vi "Begin.vi"(8 "error in":errorcluster) -> (0 "error out":errorcluster)   [LabVIEW 2023]
doc: "Called before other user functions, this VI is expected to open initial I/O refnums, load in file data, and do all program initialization. Notice that the <B>error out</B> terminal is simply used for data flow. Wiring it to other structures or subVIs ensures that this VI runs first."
uses:
  <vilib>/Rock Robotics/WPI/DriverStation/WPI_DriverStationRobotMode2.ctl
  <vilib>/Rock Robotics/WPI/Joystick/WPI_JoystickDeviceEnum.ctl
  <vilib>/Rock Robotics/WPI/RobotDrive/WPI_RobotDriveDevRef.ctl
  <vilib>/Rock Robotics/WPI/MotorControl/WPI_MotorControlDeviceRef.ctl
  <vilib>/Rock Robotics/WPI/MotorControl/WPI_MotorControlType.ctl
  <vilib>/Rock Robotics/SystemInterfaces/DIO/FPGA_DIOPWMChannel.ctl
  <vilib>/Rock Robotics/WPI/PWM/WPI_PWMDeadband.ctl
  <vilib>/Rock Robotics/SystemInterfaces/DIO/FPGA_DIOChannel.ctl
  <vilib>/Rock Robotics/WPI/SafetyOutput/WPI_SafetyOutputConfigMenu.ctl
  Robot Global Data.vi
  <vilib>/Rock Robotics/Network Tables/NT Write String Array.vi
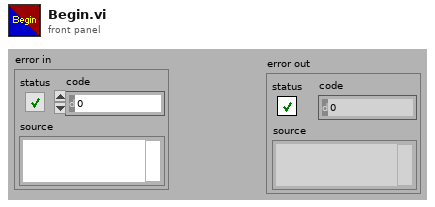
[diagram p1: front panel]
types:
  T1 = typedef "WPI_RobotDriveDevRef.ctl" = cluster{"DevStatus":errorcluster, "Motors[]":T2[], "Square Inputs":bool, "Max Output":dbl}
  T2 = typedef "WPI_MotorControlDeviceRef.ctl" = cluster{"DeviceStatus":errorcluster, "Type":T3, "PWM":cluster{"PWM Channel":T4, "DeadBand":T5}, "CAN":cluster{"Device Number":u8, "SetOutput VI Ref":variant, "GetOutput VI Ref":variant, "Enable VI Ref":variant, "Disable VI Ref":variant, "Data":variant}, "Invert":bool, "DIO PWM":cluster{"PWM \"Enable\" Channel":T4, "DIOChannel":T6, "PWM Rate":dbl}}
  T3 = typedef "WPI_MotorControlType.ctl" = enum16{"PWM", "CAN", "DIO PWM"}
  T4 = typedef "FPGA_DIOPWMChannel.ctl" = enum8{"PWM 0", "PWM 1", "PWM 2", "PWM 3", "PWM 4", "PWM 5", "PWM 6", "PWM 7", "PWM 8", "PWM 9", "PWM MXP 0", "PWM MXP 1", "PWM MXP 2", "PWM MXP 3", "PWM MXP 4", "PWM MXP 5", "PWM MXP 6", "PWM MXP 7", "PWM MXP 8", "PWM MXP 9", "Invalid"}
  T5 = typedef "WPI_PWMDeadband.ctl" = cluster{"Name":string, "maxPositivePwm":i32, "minPositivePwm":i32, "centerPwm":i32, "maxNegativePwm":i32, "minNegativePwm":i32, "angularRange":u16}
  T6 = typedef "FPGA_DIOChannel.ctl" = enum8{"DIO 0", "DIO 1", "DIO 2", "DIO 3", "DIO 4", "DIO 5", "DIO 6", "DIO 7", "DIO 8", "DIO 9", "DIO MXP 0", "DIO MXP 1", "DIO MXP 2", "DIO MXP 3", "DIO MXP 4", "DIO MXP 5", "DIO MXP 6", "DIO MXP 7", "DIO MXP 8", "DIO MXP 9", "DIO MXP 10", "DIO MXP 11", "DIO MXP 12", "DIO MXP 13", "DIO MXP 14", "DIO MXP 15", "SPI Port CS1", "SPI Port CS2", "SPI Port CS3", "SPI Port MISO", "SPI Port MOSI", "Invalid"}
  T7 = typedef "WPI_SafetyOutputConfigMenu.ctl" = enum16{"Enable", "Disable"}
  T8 = typedef "WPI_JoystickDeviceEnum.ctl" = enum16{"USB 0", "USB 1", "USB 2", "USB 3", "USB 4", "USB 5"}
  T9 = typedef "WPI_DriverStationRobotMode2.ctl" = enum16{"Autonomous Disabled", "Autonomous Enabled", "Teleop Disabled", "Teleop Enabled", "Disconnected", "Finish", "Test Disabled", "Test Enabled", "Emergency Stopped"}
  T10 = typedef "WPI_JoystickDevRef.ctl" = cluster{"Device":T8}
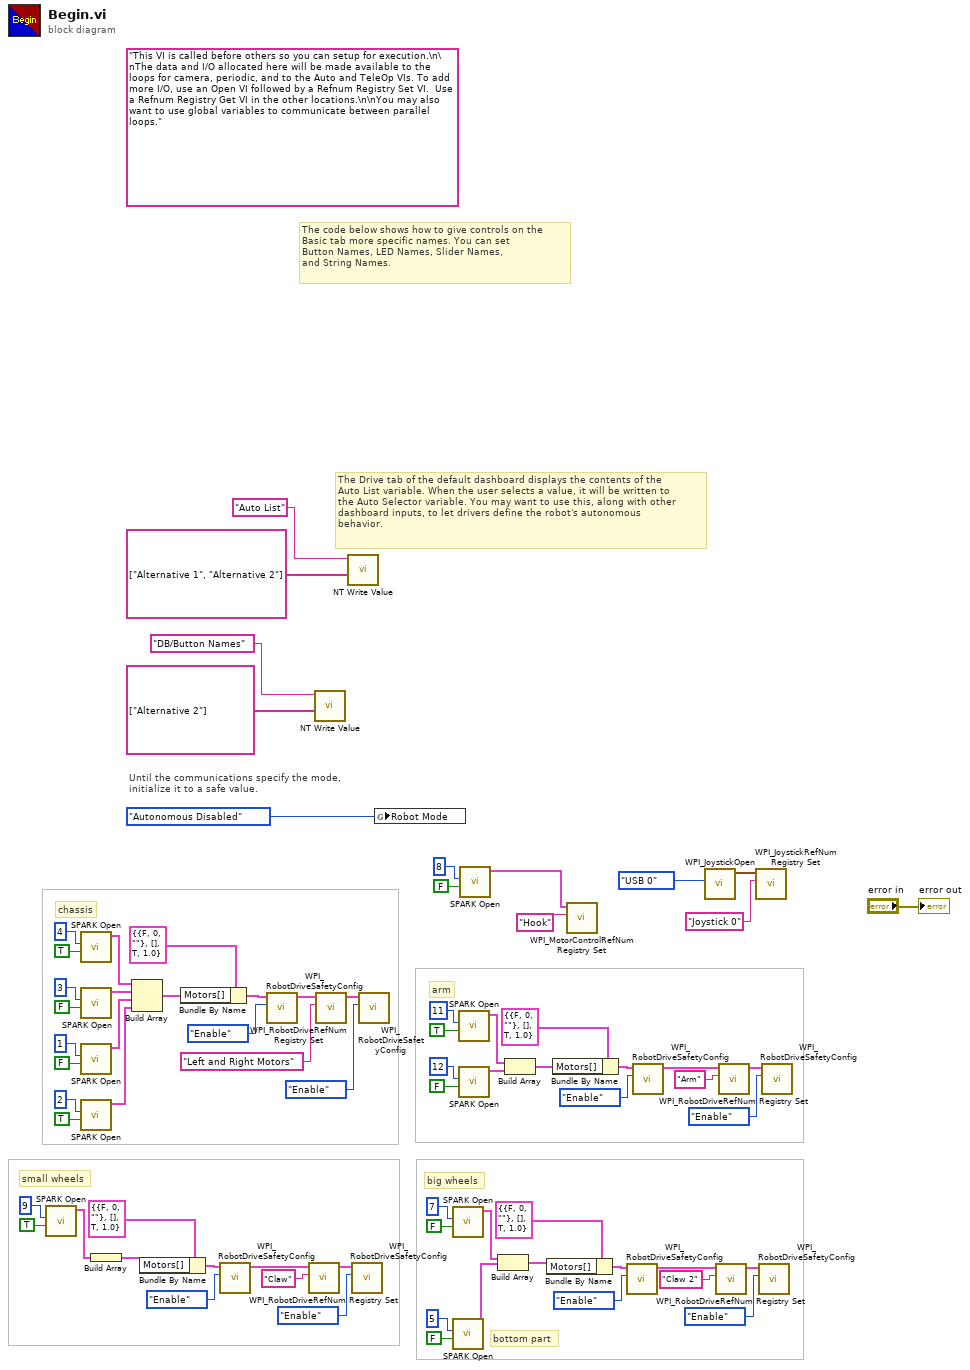
[diagram p0: block diagram]
diagram:
  (unwired) "This VI is called before others so you can setup for execution.\n\nThe data and I/O allocated here will be made available to the loops for camera, periodic, and to the Auto and TeleOp VIs. To add more I/O, use an Open VI followed by a Refnum Registry Set VI.  Use a Refnum Registry Get VI in the other locations.\n\nYou may also want to use global variables to communicate between parallel loops."
  # "bottom part"
  # "arm"
  # "small wheels"
  # "big wheels"
  # "chassis"
  # "The Drive tab of the default dashboard displays the contents of the\nAuto List variable. When the user selects a value, it will be written to\nthe Auto Selector variable. You may want to use this, along with other\ndashboard inputs, to let drivers define the robot's autonomous\nbehavior."
  # "The code below shows how to give controls on the\nBasic tab more specific names. You can set\nButton Names, LED Names, Slider Names,\nand String Names."
  # "Until the communications specify the mode,\ninitialize it to a safe value."
  n1 = call <vilib>:"SPARK Open.vi"("Invert"=TRUE, "Device Number"=u8 9) -> ("MotorControlDeviceRef"=w38:T2)  [unwired: 8 in, 1 out]
  n2 = call <vilib>:"SPARK Open.vi"("Invert"=TRUE, "Device Number"=u8 4) -> ("MotorControlDeviceRef"=w52:T2)  [unwired: 8 in, 1 out]
  n3 = call <vilib>:"SPARK Open.vi"("Invert"=FALSE, "Device Number"=u8 3) -> ("MotorControlDeviceRef"=w50:T2)  [unwired: 8 in, 1 out]
  n4 = call <vilib>:"SPARK Open.vi"("Invert"=FALSE, "Device Number"=u8 1) -> ("MotorControlDeviceRef"=w51:T2)  [unwired: 8 in, 1 out]
  n5 = call <vilib>:"SPARK Open.vi"("Invert"=TRUE, "Device Number"=u8 2) -> ("MotorControlDeviceRef"=w49:T2)  [unwired: 8 in, 1 out]
  n6 = Build Array(w38) -> (w34:T2[])
  n7 = Build Array(w52, w50, w51, w49) -> (w45:T2[])
  n8 = Bundle By Name(cluster=T1 {"DevStatus"={"status"=FALSE, "code"=0, "source"=""}, "Motors[]"=[], "Square Inputs"=TRUE, "Max Output"=1.0} ("RobotDriveDevRef"), "Motors[]"=w34) -> (w37:T1)
  n9 = Bundle By Name(cluster=T1 {"DevStatus"={"status"=FALSE, "code"=0, "source"=""}, "Motors[]"=[], "Square Inputs"=TRUE, "Max Output"=1.0} ("RobotDriveDevRef"), "Motors[]"=w45) -> (w48:T1)
  n10 = call <vilib>:"WPI_RobotDriveSafetyConfig.vi"("mode"=WPI_SafetyOutputConfigMenu."Enable", "RobotDriveDevRef"=w37) -> ("RobotDriveDevRef"=w33:T1)  [unwired: 2 in, 7 out]
  n11 = call <vilib>:"WPI_RobotDriveSafetyConfig.vi"("mode"=WPI_SafetyOutputConfigMenu."Enable", "RobotDriveDevRef"=w48) -> ("RobotDriveDevRef"=w44:T1)  [unwired: 2 in, 7 out]
  n12 = call <vilib>:"WPI_RobotDriveRefNum Registry Set.vi"("refnum name"="Claw", "RobotDriveDevRef"=w33) -> ("RobotDriveDevRef"=w42:T1)  [unwired: 2 in, 7 out]
  n13 = call-poly <vilib>:"NT Write Value.vi"("value"=string[] ["Alternative 2"], "name"="DB/Button Names" ("Name")) -> ()  [unwired: 9 in, 1 out]
  n14 = call <vilib>:"WPI_RobotDriveRefNum Registry Set.vi"("refnum name"="Left and Right Motors", "RobotDriveDevRef"=w44) -> ("RobotDriveDevRef"=w71:T1)  [unwired: 2 in, 7 out]
  n15 = call-poly <vilib>:"NT Write Value.vi"("value"=string[] ["Alternative 1", "Alternative 2"] ("String Array"), "name"="Auto List" ("Name")) -> ()  [unwired: 9 in, 1 out]
  n16 = call <vilib>:"WPI_RobotDriveSafetyConfig.vi"("mode"=WPI_SafetyOutputConfigMenu."Enable", "RobotDriveDevRef"=w42) -> ()  [unwired: 8 in, 2 out]
  n17 = call <vilib>:"WPI_RobotDriveSafetyConfig.vi"("mode"=WPI_SafetyOutputConfigMenu."Enable", "RobotDriveDevRef"=w71) -> ()  [unwired: 8 in, 2 out]
  n18 = global write "Robot Global Data.vi" "Robot Mode"(WPI_DriverStationRobotMode2."Autonomous Disabled" ("Robot Mode")) -> ()
  n19 = call <vilib>:"SPARK Open.vi"("Invert"=FALSE, "Device Number"=u8 7) -> ("MotorControlDeviceRef"=w13:T2)  [unwired: 8 in, 1 out]
  n20 = call <vilib>:"SPARK Open.vi"("Invert"=FALSE, "Device Number"=u8 5) -> ("MotorControlDeviceRef"=w6:T2)  [unwired: 8 in, 1 out]
  n21 = call <vilib>:"SPARK Open.vi"("Invert"=TRUE, "Device Number"=u8 11) -> ("MotorControlDeviceRef"=w25:T2)  [unwired: 8 in, 1 out]
  n22 = call <vilib>:"SPARK Open.vi"("Invert"=FALSE, "Device Number"=u8 12) -> ("MotorControlDeviceRef"=w24:T2)  [unwired: 8 in, 1 out]
  n23 = call <vilib>:"SPARK Open.vi"("Invert"=FALSE, "Device Number"=u8 8) -> ("MotorControlDeviceRef"=w1:T2)  [unwired: 8 in, 1 out]
  n24 = Build Array(w13, w6) -> (w9:T2[])
  n25 = Build Array(w25, w24) -> (w20:T2[])
  n26 = Bundle By Name(cluster=T1 {"DevStatus"={"status"=FALSE, "code"=0, "source"=""}, "Motors[]"=[], "Square Inputs"=TRUE, "Max Output"=1.0} ("RobotDriveDevRef"), "Motors[]"=w9) -> (w12:T1)
  n27 = Bundle By Name(cluster=T1 {"DevStatus"={"status"=FALSE, "code"=0, "source"=""}, "Motors[]"=[], "Square Inputs"=TRUE, "Max Output"=1.0} ("RobotDriveDevRef"), "Motors[]"=w20) -> (w23:T1)
  n28 = call <vilib>:"WPI_MotorControlRefNum Registry Set.vi"("refnum name"="Hook", "MotorControlDevRef"=w1) -> ()  [unwired: 8 in, 2 out]
  n29 = call <vilib>:"WPI_RobotDriveSafetyConfig.vi"("mode"=WPI_SafetyOutputConfigMenu."Enable", "RobotDriveDevRef"=w12) -> ("RobotDriveDevRef"=w8:T1)  [unwired: 2 in, 7 out]
  n30 = call <vilib>:"WPI_RobotDriveSafetyConfig.vi"("mode"=WPI_SafetyOutputConfigMenu."Enable", "RobotDriveDevRef"=w23) -> ("RobotDriveDevRef"=w19:T1)  [unwired: 2 in, 7 out]
  n31 = call <vilib>:"WPI_JoystickOpen.vi"("JoystickDevice"=WPI_JoystickDeviceEnum."USB 0") -> ("JoystickDevRef"=w67:T10)  [unwired: 10 in]
  n32 = call <vilib>:"WPI_RobotDriveRefNum Registry Set.vi"("refnum name"="Claw 2", "RobotDriveDevRef"=w8) -> ("RobotDriveDevRef"=w17:T1)  [unwired: 2 in, 7 out]
  n33 = call <vilib>:"WPI_RobotDriveRefNum Registry Set.vi"("refnum name"="Arm", "RobotDriveDevRef"=w19) -> ("RobotDriveDevRef"=w31:T1)  [unwired: 2 in, 7 out]
  n34 = call <vilib>:"WPI_JoystickRefNum Registry Set.vi"("refnum name"="Joystick 0", "JoystickDevRef"=w67) -> ()  [unwired: 8 in, 2 out]
  n35 = call <vilib>:"WPI_RobotDriveSafetyConfig.vi"("mode"=WPI_SafetyOutputConfigMenu."Enable", "RobotDriveDevRef"=w17) -> ()  [unwired: 8 in, 2 out]
  n36 = call <vilib>:"WPI_RobotDriveSafetyConfig.vi"("mode"=WPI_SafetyOutputConfigMenu."Enable", "RobotDriveDevRef"=w31) -> ()  [unwired: 8 in, 2 out]
  "error out" <- "error in"
